vi "sendParameter2SV.vi"(0 "Connection In":string, 1 "Parameter":variant, 2 "typeDescriptor":string, 3 "ms timeout (0)":i32, 5 "error in (no error)":errorcluster) -> (14 "connection out":string, 16 "timed out":bool, 19 "error out":errorcluster)   [LabVIEW 2012, in "HGF_SV.lvlib"]
doc: "Sends parameters to a shared variable after converting them to variant and adding the type descriptor. This can be used to test the SV-Class, especially the monitoring class."
uses:
  HGF_SV.lvlib
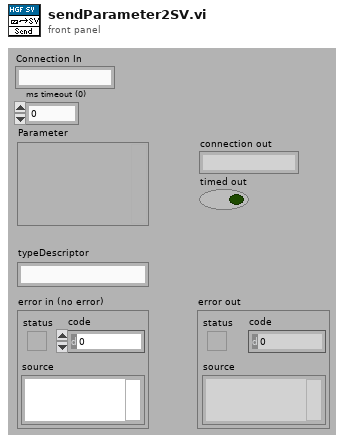
[diagram p1: front panel]
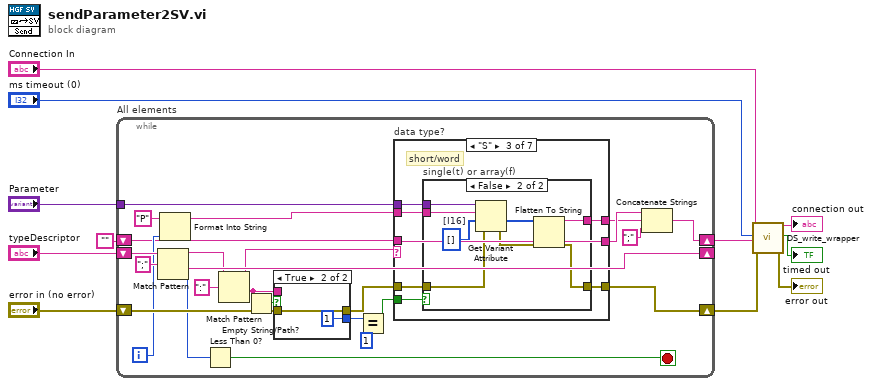
[diagram p0: block diagram]
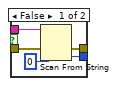
[diagram p2: hidden frame]
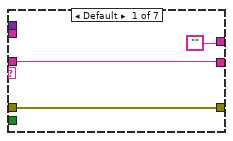
[diagram p3: hidden frame]
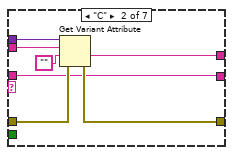
[diagram p4: hidden frame]
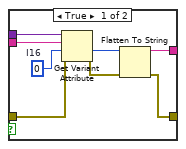
[diagram p5: hidden frame]
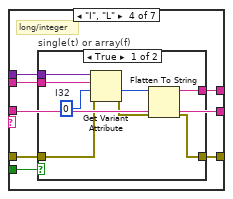
[diagram p6: hidden frame]
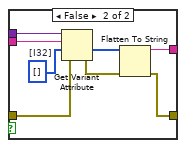
[diagram p7: hidden frame]
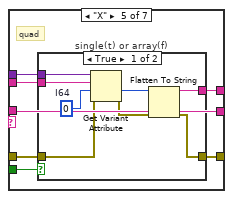
[diagram p8: hidden frame]
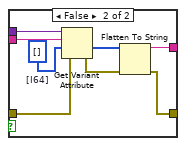
[diagram p9: hidden frame]
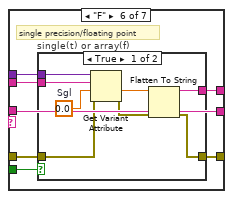
[diagram p10: hidden frame]
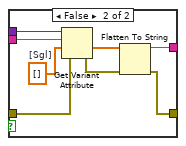
[diagram p11: hidden frame]
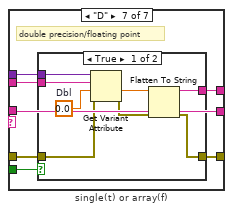
[diagram p12: hidden frame]
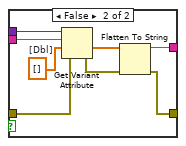
[diagram p13: hidden frame]
diagram:
  n1 = while "All elements" {
    shift-right: [w33] -> _
    shift-left: "typeDescriptor" -> [w35]
    shift-right: [w23] -> w6
    shift-left: "error in (no error)" -> [w36]
    tunnel: "Parameter" -> [w22]
    shift-right: [w17] -> w7
    shift-left: "" -> [w18]
    i -> [w27]
    stop <- w32 stop-if-true
    n2 = Match Pattern(string=w35, regular expression=";") -> (before substring=w30:string, after substring=w33:string, offset past match=w31:i32)  [unwired: 2 out]
    n3 = Format Into String(initial string="P", w27) -> (resulting string=w26:string)  [unwired: 2 in, 1 out]
    n4 = Less Than 0?(x=w31) -> (x < 0?=w32:bool)
    n5 = Match Pattern(string=w30, regular expression=":") -> (before substring=w25:string, after substring=w12:string)  [unwired: 3 out]
    n6 = Empty String/Path?(string/path=w12) -> (empty?=w13:bool)
    n7 = case shown="True" w13 {
      tunnel: w12 -> [w40 _]
      tunnel: w36 -> [w39 w43]
      tunnel: [w38 w43] -> w24
      tunnel: [w37 1 ("default value 1")] -> w21
      frame False {
        n8 = Scan From String(input string=w40, error in=w39, default 1=0 ("default value 1")) -> (error out=w38:errorcluster, output 1=w37:i32)  [unwired: 2 in, 2 out]
      }
      frame True {
      }
    }
    n9 = Equal?(x=w21, y=1) -> (x = y?=w19:bool)
    n10 = case "data type?" shown="\"S\"" w25 {
      tunnel: w26 -> [_ w51 w58 w81 w104 w127 w150]
      tunnel: w24 -> [w46 w52 w59 w82 w105 w128 w151]
      tunnel: [w46 w49 w57 w80 w103 w126 w149] -> w23
      tunnel: w22 -> [_ w53 w60 w83 w106 w129 w152]
      tunnel: w19 -> [_ _ w56 w79 w102 w125 w148]
      tunnel: [w45 w48 w54 w77 w100 w123 w146] -> w16
      tunnel: w18 -> [w45 w48 w54 w77 w100 w123 w146]
      tunnel: ["" w47 w55 w78 w101 w124 w147] -> w15
      frame Default {
      }
      frame "C" {
        n11 = Get Variant Attribute(Variant=w53, name=w51, default value (empty Variant)="", error in=w52) -> (value=w47:string, error out=w49:errorcluster)  [unwired: 2 out]
      }
      frame "S" {
        # "short/word"
        n12 = case "single(t) or array(f)" shown="False" w56 {
          tunnel: w60 -> [w68 w76]
          tunnel: w59 -> [w67 w75]
          tunnel: w58 -> [w66 w74]
          tunnel: [w63 w69] -> w57
          tunnel: [w62 w72] -> w55
          frame True {
            w65 = i16 0  # I16
            n13 = Get Variant Attribute(Variant=w68, name=w66, default value (empty Variant)=w65, error in=w67) -> (value=w61:i16, error out=w64:errorcluster)  [unwired: 2 out]
            n14 = Flatten To String(anything=w61, error in (no error)=w64) -> (data string=w62:string, error out=w63:errorcluster)  [unwired: 3 out]
          }
          frame False {
            w73 = i16[] []  # [I16]
            n15 = Get Variant Attribute(Variant=w76, name=w74, default value (empty Variant)=w73, error in=w75) -> (value=w71:i16[], error out=w70:errorcluster)  [unwired: 2 out]
            n16 = Flatten To String(anything=w71, error in (no error)=w70) -> (data string=w72:string, error out=w69:errorcluster)  [unwired: 3 out]
          }
        }
      }
      frame "I", "L" {
        # "long/integer"
        n17 = case "single(t) or array(f)" shown="True" w79 {
          tunnel: w83 -> [w91 w99]
          tunnel: w82 -> [w90 w98]
          tunnel: w81 -> [w89 w97]
          tunnel: [w86 w92] -> w80
          tunnel: [w85 w95] -> w78
          frame True {
            w88 = 0  # I32
            n18 = Get Variant Attribute(Variant=w91, name=w89, default value (empty Variant)=w88, error in=w90) -> (value=w84:i32, error out=w87:errorcluster)  [unwired: 2 out]
            n19 = Flatten To String(anything=w84, error in (no error)=w87) -> (data string=w85:string, error out=w86:errorcluster)  [unwired: 3 out]
          }
          frame False {
            w96 = i32[] []  # [I32]
            n20 = Get Variant Attribute(Variant=w99, name=w97, default value (empty Variant)=w96, error in=w98) -> (value=w94:i32[], error out=w93:errorcluster)  [unwired: 2 out]
            n21 = Flatten To String(anything=w94, error in (no error)=w93) -> (data string=w95:string, error out=w92:errorcluster)  [unwired: 3 out]
          }
        }
      }
      frame "X" {
        # "quad"
        n22 = case "single(t) or array(f)" shown="True" w102 {
          tunnel: w106 -> [w114 w122]
          tunnel: w105 -> [w113 w121]
          tunnel: w104 -> [w112 w120]
          tunnel: [w109 w115] -> w103
          tunnel: [w108 w118] -> w101
          frame True {
            w111 = i64 0  # I64
            n23 = Get Variant Attribute(Variant=w114, name=w112, default value (empty Variant)=w111, error in=w113) -> (value=w107:i64, error out=w110:errorcluster)  [unwired: 2 out]
            n24 = Flatten To String(anything=w107, error in (no error)=w110) -> (data string=w108:string, error out=w109:errorcluster)  [unwired: 3 out]
          }
          frame False {
            w119 = i64[] []  # [I64]
            n25 = Get Variant Attribute(Variant=w122, name=w120, default value (empty Variant)=w119, error in=w121) -> (value=w117:i64[], error out=w116:errorcluster)  [unwired: 2 out]
            n26 = Flatten To String(anything=w117, error in (no error)=w116) -> (data string=w118:string, error out=w115:errorcluster)  [unwired: 3 out]
          }
        }
      }
      frame "F" {
        # "single precision/floating point"
        n27 = case "single(t) or array(f)" shown="True" w125 {
          tunnel: w129 -> [w137 w145]
          tunnel: w128 -> [w136 w144]
          tunnel: w127 -> [w135 w143]
          tunnel: [w132 w138] -> w126
          tunnel: [w131 w141] -> w124
          frame True {
            w134 = sgl 0.0  # Sgl
            n28 = Get Variant Attribute(Variant=w137, name=w135, default value (empty Variant)=w134, error in=w136) -> (value=w130:sgl, error out=w133:errorcluster)  [unwired: 2 out]
            n29 = Flatten To String(anything=w130, error in (no error)=w133) -> (data string=w131:string, error out=w132:errorcluster)  [unwired: 3 out]
          }
          frame False {
            w142 = sgl[] []  # [Sgl]
            n30 = Get Variant Attribute(Variant=w145, name=w143, default value (empty Variant)=w142, error in=w144) -> (value=w140:sgl[], error out=w139:errorcluster)  [unwired: 2 out]
            n31 = Flatten To String(anything=w140, error in (no error)=w139) -> (data string=w141:string, error out=w138:errorcluster)  [unwired: 3 out]
          }
        }
      }
      frame "D" {
        # "double precision/floating point"
        n32 = case "single(t) or array(f)" shown="True" w148 {
          tunnel: w152 -> [w160 w168]
          tunnel: w151 -> [w159 w167]
          tunnel: w150 -> [w158 w166]
          tunnel: [w155 w161] -> w149
          tunnel: [w154 w164] -> w147
          frame True {
            w157 = 0.0  # Dbl
            n33 = Get Variant Attribute(Variant=w160, name=w158, default value (empty Variant)=w157, error in=w159) -> (value=w153:dbl, error out=w156:errorcluster)  [unwired: 2 out]
            n34 = Flatten To String(anything=w153, error in (no error)=w156) -> (data string=w154:string, error out=w155:errorcluster)  [unwired: 3 out]
          }
          frame False {
            w165 = dbl[] []  # [Dbl]
            n35 = Get Variant Attribute(Variant=w168, name=w166, default value (empty Variant)=w165, error in=w167) -> (value=w163:dbl[], error out=w162:errorcluster)  [unwired: 2 out]
            n36 = Flatten To String(anything=w163, error in (no error)=w162) -> (data string=w164:string, error out=w161:errorcluster)  [unwired: 3 out]
          }
        }
      }
    }
    n37 = Concatenate Strings(w16, w15, ";" ("string")) -> (w17:string)
  }
  n38 = call "DS_write_wrapper.vi"("Connection In"="Connection In", "ms timeout (0)"="ms timeout (0)", "rawData"=w7, "error in"=w6) -> ("connection out"=→"connection out":string, "timed out"=→"timed out":bool, "error out"=→"error out":errorcluster)  [unwired: 13 out]
